vi "ValueConvert.vi"(10 "ValueIn":T1, 11 "MotorType":T2) -> (2 "FilteredValue":T1, 3 "CANBusData":u8[](array[numeric]) format="%x")   [LabVIEW 2019, in "CubeMarsBLDClib.lvlib"]
uses:
  CubeMarsBLDClib.lvlib
  MotorParameters.ctl
  MotorType.ctl
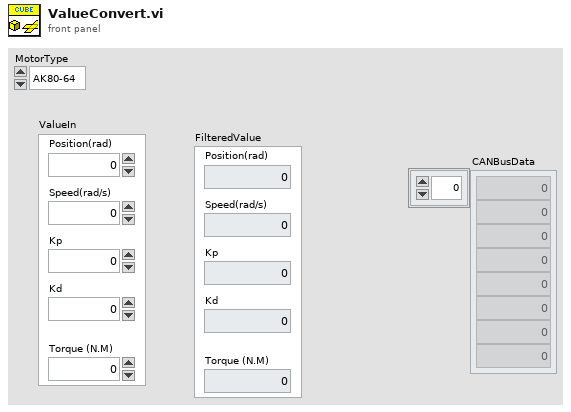
[diagram p1: front panel]
types:
  T1 = typedef "CubeMarsBLDClib.lvlib/MotorParameters.ctl" = cluster{"Position(rad)":dbl, "Speed(rad/s)":dbl, "Kp":dbl, "Kd":dbl, "Torque (N.M)":dbl}
  T2 = typedef "CubeMarsBLDClib.lvlib/MotorType.ctl" = enum16{"AK80-64", "AK80-9", "AK80-8", "AK80-6", "AK70-10", "AK60-6", "AK10-9"}
  T3 = cluster{"Position(rad)":u16, "Speed(rad/s)":u16, "Kp":u16, "Kd":u16, "Torque (N.M)":u16}
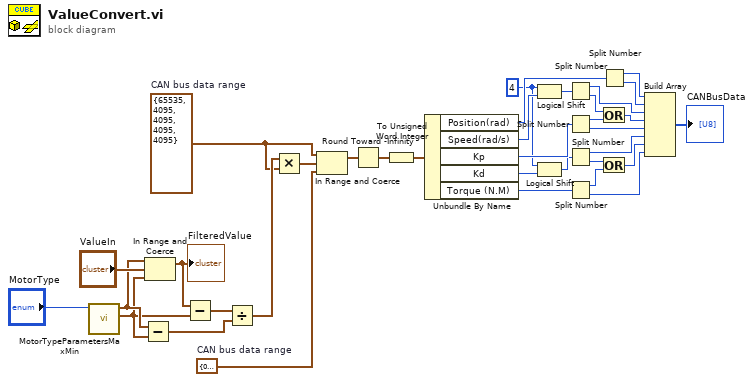
[diagram p0: block diagram]
diagram:
  w5 = i16 4 ("y")
  w26 = T3 {"Position(rad)"=0, "Speed(rad/s)"=0, "Kp"=0, "Kd"=0, "Torque (N.M)"=0}  # CAN bus data range
  w27 = T3 {"Position(rad)"=65535, "Speed(rad/s)"=4095, "Kp"=4095, "Kd"=4095, "Torque (N.M)"=4095}  # CAN bus data range
  n1 = call "MotorTypeParametersMaxMin.vi"("MotorType"="MotorType") -> ("Min"=w31:T1, "Max"=w32:T1)  [unwired: 9 in]
  n2 = Subtract(x=w32, y=w31) -> (x-y=w30:T1)
  n3 = In Range and Coerce(upper limit=w32, x="ValueIn", lower limit=w31) -> (coerced(x)=w33:T1)  [unwired: 1 out]
  "FilteredValue" <- w33
  n4 = Subtract(x=w33, y=w31) -> (x-y=w29:T1)
  n5 = Divide(x=w29, y=w30) -> (x/y=w28:T1)
  n6 = Multiply(x=w28, y=w27) -> (x*y=w25:T1)
  n7 = In Range and Coerce(upper limit=w27, x=w25, lower limit=w26) -> (coerced(x)=w24:T1)  [unwired: 1 out]
  n8 = Round Toward -Infinity(1:w24) -> (0:w23:T1)
  n9 = To Unsigned Word Integer(number=w23) -> (unsigned 16bit integer=w22:T3)
  n10 = Unbundle By Name(w22) -> ("Position(rad)"=w21:u16, "Speed(rad/s)"=w14:u16, "Kp"=w18:u16, "Kd"=w7:u16, "Torque (N.M)"=w17:u16)
  n11 = Logical Shift(y=w5, x=w14) -> (x << y=w13:u16)
  n12 = Logical Shift(y=w5, x=w7) -> (x << y=w6:u16)
  n13 = Split Number(x=w13) -> (hi(x)=w16:u8, lo(x)=w12:u8)
  n14 = Split Number(x=w18) -> (hi(x)=w11:u8, lo(x)=w15:u8)
  n15 = Split Number(x=w6) -> (hi(x)=w9:u8, lo(x)=w4:u8)
  n16 = Split Number(x=w17) -> (hi(x)=w3:u8, lo(x)=w8:u8)
  n17 = Or(x=w12, y=w11) -> (x .or. y?=w10:u8)
  n18 = Or(x=w4, y=w3) -> (x .or. y?=w2:u8)
  n19 = Split Number(x=w21) -> (hi(x)=w20:u8, lo(x)=w19:u8)
  n20 = Build Array(w20, w19, w16, w10, w15, w9, w2, w8) -> (→"CANBusData":u8[])
